vi "Read Network Protocol.vi"(8 "error in (no error)":errorcluster, 11 "Modbus API in":refnum<class "Modbus API.lvclass">) -> (0 "error out":errorcluster, 2 "Network Protocol":refnum<class "Network Protocol.lvclass">, 3 "Modbus API out":refnum<class "Modbus API.lvclass">)   [LabVIEW 2021, in "Modbus API.lvclass"]
uses:
  Modbus API.lvclass
  Network Protocol/Network Protocol.lvclass
  Modbus API.lvclass/Modbus API.ctl
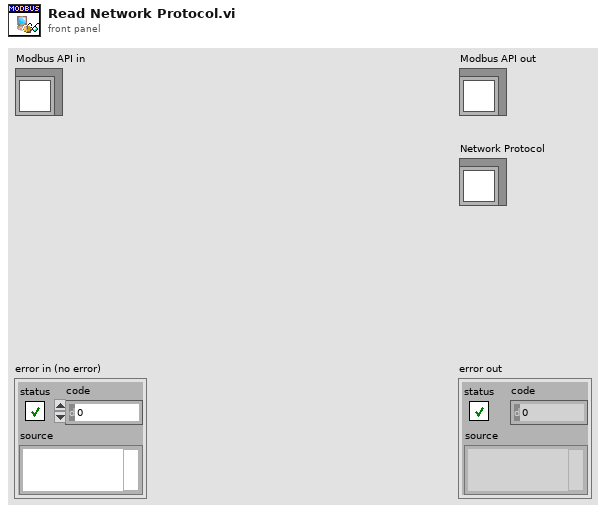
[diagram p1: front panel]
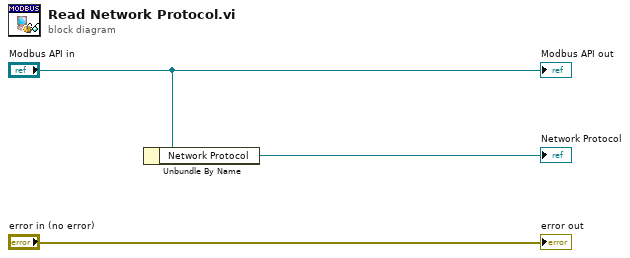
[diagram p0: block diagram]
diagram:
  n1 = Unbundle By Name("Modbus API in") -> ("Network Protocol"=→"Network Protocol":refnum<class "Network Protocol.lvclass">)
  "error out" <- "error in (no error)"
  "Modbus API out" <- "Modbus API in"
